vi "Simulated Excitation.vi"() -> (0 "Analog Input":i16)   [LabVIEW 2010]
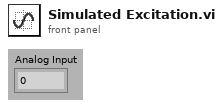
[diagram p1: front panel]
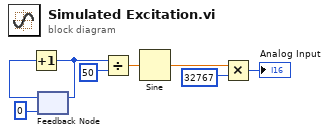
[diagram p0: block diagram]
diagram:
  n1 = feedback #1(0) -> (w3:i32)
  n2 = Increment(x=w3) -> (x+1=w4:i32)
  n3 = feedback-in #1(w4) -> ()
  n4 = Divide(x=w4, y=50) -> (x/y=w6:dbl)
  n5 = Sine(x=w6) -> (sin(x)=w2:dbl)
  n6 = Multiply(x=w2, y=i16 32767) -> (x*y=→"Analog Input":i16)
